vi "LoadModel.vi"(8 "error in (no error)":errorcluster, 10 "Actor In":refnum<class "Actor.lvclass">, 11 "GRMActor in":refnum<class "LaserController.lvclass">) -> (0 "error out":errorcluster, 3 "GRMActor out":refnum<class "LaserController.lvclass">)   [LabVIEW 2020, in "LaserController.lvlib" / "LaserController.lvclass"]
uses:
  LaserController.lvclass
  <vilib>/ActorFramework/Actor/Actor.lvclass
  Model/Hardware Layer/Simulation Hardware/DemoLasers/DemoLasers/DemoLasers.lvclass
  C:/Program Files/National Instruments/LabVIEW 2020/vi.lib/ActorFramework/Actor/Actor.lvclass
  Model/Hardware Abstraction Layer/Component/GenericActor/GenericActor/GenericController.lvclass
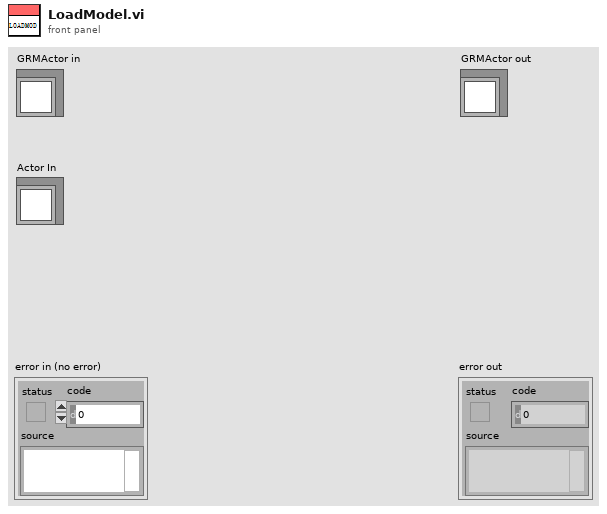
[diagram p1: front panel]
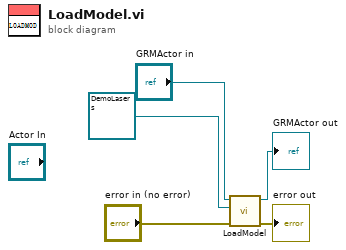
[diagram p0: block diagram]
diagram:
  n1 = call-parent "LoadModel.vi"("error in (no error)"="error in (no error)", "Actor In"=refnum<class "DemoLasers.lvclass"> refnum ("DemoLasers.lvlib:DemoLasers.lvclass"), "GRMActor in"="GRMActor in") -> ("error out"=→"error out":errorcluster, "GRMActor out"=→"GRMActor out":refnum<class "LaserController.lvclass">)  [unwired: 7 in]
